vi "MPM_Get_Read_Range_Mode.vi"(8 "error in (no error)":errorcluster, 11 ".NET Reference in":refnum<k24>) -> (0 "error out":errorcluster, 1 "mode":enum16{"Manual", "Auto"}(ring), 3 "Reference out":refnum<k24>)   [LabVIEW 2017]
uses:
  C:/Users/Ssantec_Test/Documents/Instrument_DLL_Sample_Labview_20250826_Ver1.5.0_x64/DLL/InstrumentDLL.dll
  DLL/InstrumentDLL.dll
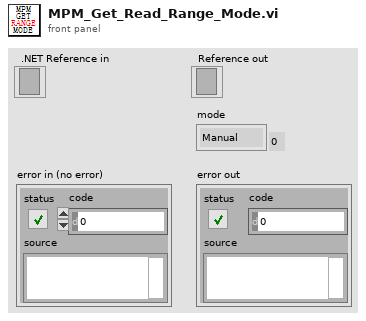
[diagram p1: front panel]
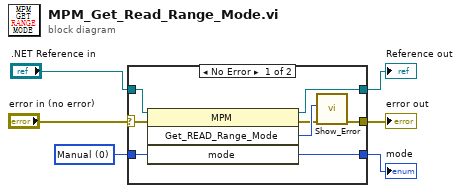
[diagram p0: block diagram]
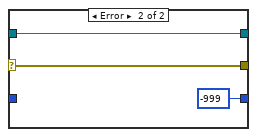
[diagram p2: hidden frame]
diagram:
  w4 = 0 items=["Manual", "Auto"] ("mode")
  n1 = case shown="No Error" "error in (no error)" {
    selector: "error in (no error)" -> [w10 w17]
    tunnel: [w14 w16] -> w6
    tunnel: ".NET Reference in" -> [w13 w16]
    tunnel: w4 -> [w12 _]
    tunnel: [w7 w17] -> w3
    tunnel: [w11 -999 ("mode")] -> w2
    frame No Error {
      n2 = invoke on="调用节点" class="MPM" method="Get_READ_Range_Mode"(reference=w13, error in=w10, "mode"=w12) -> (reference out=w14:refnum<k24>, error out=w8:errorcluster, "Get_READ_Range_Mode"=w9:i32, "mode"=w11:i32)  [unwired: 1 in]
      n3 = call "Show_Error.vi"("error in (no error)"=w8, "Error"=w9) -> ("error out"=w7:errorcluster)  [unwired: 9 in]
    }
    frame Error {
    }
  }
  "Reference out" <- w6
  "error out" <- w3
  "mode" <- w2
